vi "Get Instrument Info.vi"(0 "Power Meter Base in":refnum<class "Power Meter Base.lvclass">, 11 "error in (no error)":errorcluster) -> (4 "Power Meter Base out":refnum<class "Power Meter Base.lvclass">, 15 "error out":errorcluster)   [LabVIEW 2023, in "RFFixtureCharact.Instruments.lvlib" / "Power Meter Base.lvclass"]
uses:
  Power Meter Base.lvclass
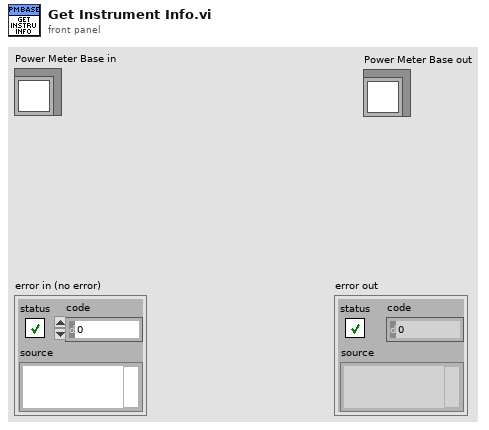
[diagram p1: front panel]
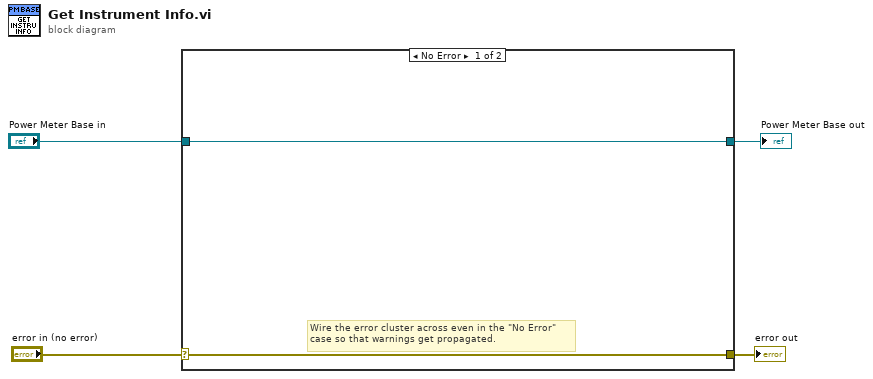
[diagram p0: block diagram]
diagram:
  n1 = case shown="No Error" "error in (no error)" {
    selector: "error in (no error)" -> [w5 w8]
    tunnel: [w5 w8] -> w3
    tunnel: [w6 w7] -> w1
    tunnel: "Power Meter Base in" -> [w6 w7]
    frame No Error {
      # "Wire the error cluster across even in the \"No Error\"\ncase so that warnings get propagated."
    }
    frame Error {
    }
  }
  "error out" <- w3
  "Power Meter Base out" <- w1
